vi "Write Group.vi"(8 "error in (no error)":errorcluster, 10 "Group":string, 11 "bt_Blackboard_Leaf Type in":refnum<class "bt_Blackboard_Leaf Type.lvclass">) -> (0 "error out":errorcluster, 3 "bt_Blackboard_Leaf Type out":refnum<class "bt_Blackboard_Leaf Type.lvclass">)   [LabVIEW 2021, in "BT.lvlib" / "bt_Blackboard_Leaf Type.lvclass"]
uses:
  bt_Blackboard_Leaf Type.lvclass
  bt_Blackboard_Leaf Type.lvclass/bt_Blackboard_Leaf Type.ctl
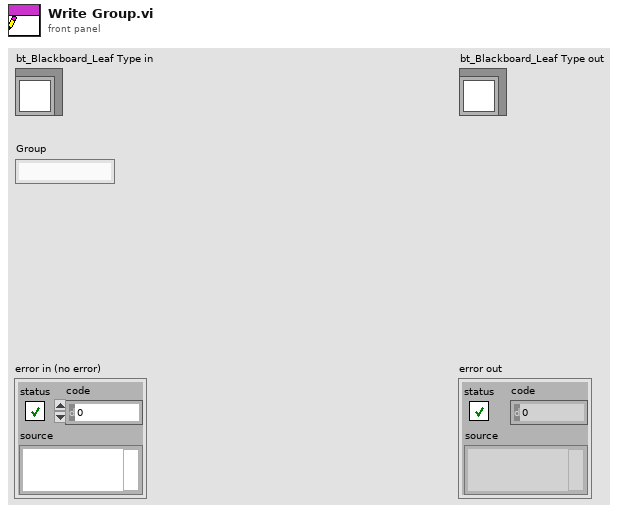
[diagram p1: front panel]
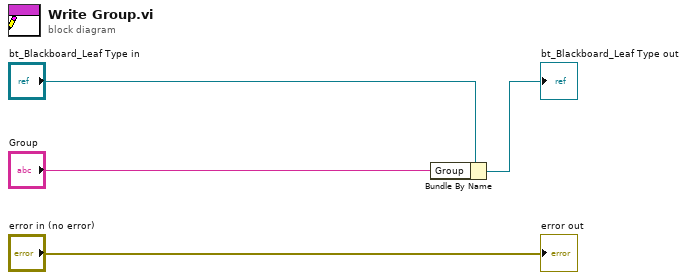
[diagram p0: block diagram]
diagram:
  n1 = Bundle By Name(cluster="bt_Blackboard_Leaf Type in", "Group"="Group") -> (→"bt_Blackboard_Leaf Type out":refnum<class "bt_Blackboard_Leaf Type.lvclass">)
  "error out" <- "error in (no error)"
